vi "DataBase.vi"(7 "udl名称":string="access.udl", 9 "parameters":T1[](array[typedef]), 11 "SQL query":string) -> (1 "recordset data":variant[][](array[variant]))   [LabVIEW 2012]
uses:
  <vilib>/addons/database/Auxilliary.llb/DB Tools Parameter Info.ctl
  <vilib>/addons/database/Auxilliary.llb/DB Tools DataTypes.ctl
  <vilib>/addons/database/Auxilliary.llb/DB Tools Parameter Dir.ctl
  <vilib>/addons/database/Connection.llb/DB Tools Open Connec (Path).vi
  <vilib>/addons/database/Command.llb/Cmd Execute.vi
  <vilib>/addons/database/Recordset.llb/Rec Fetch Recordset Data (CR).vi
  <vilib>/addons/database/Recordset.llb/Rec Destroy - Command.vi
  <vilib>/addons/database/Command.llb/Cmd Delete.vi
  <vilib>/addons/database/NI_Database_API.lvlib
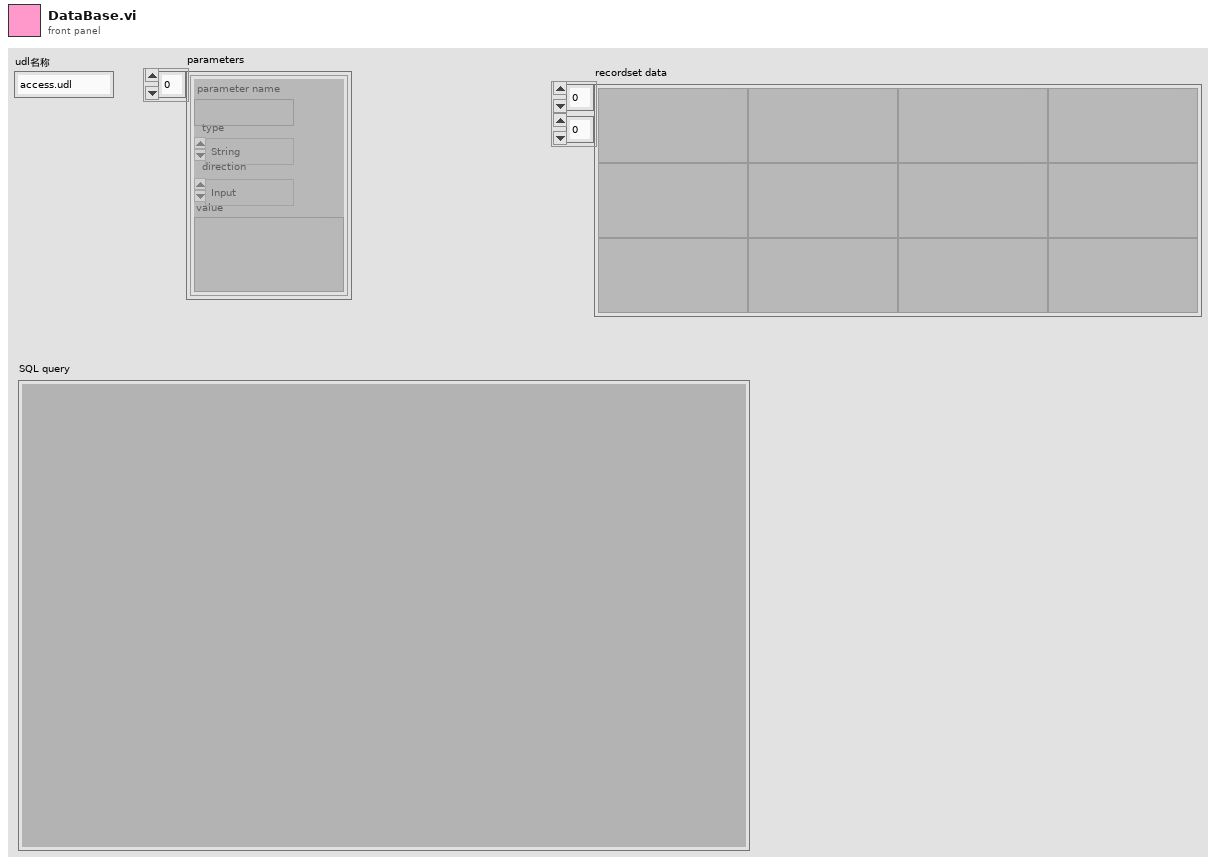
[diagram p1: front panel]
types:
  T1 = typedef "NI_Database_API.lvlib/DB Tools Parameter Info.ctl" = cluster{"parameter name":string, "type":T2, "direction":T3, "value":variant}
  T2 = typedef "NI_Database_API.lvlib/DB Tools DataTypes.ctl" = enum16{"String", "Long (I32)", "Single (SGL)", "Double (DBL)", "Date/Time", "Binary"}
  T3 = typedef "NI_Database_API.lvlib/DB Tools Parameter Dir.ctl" = enum32{"Input", "Output", "Input/Output", "Return Value"}
  T4 = typedef "NI_Database_API.lvlib/Conn ObjectReference.ctl" = refnum<k1>
  T5 = typedef "NI_Database_API.lvlib/Cmd ObjectReference.ctl" = refnum<k1>
  T6 = typedef "NI_Database_API.lvlib/Cmd-Rec Object Reference.ctl" = refnum<k1>
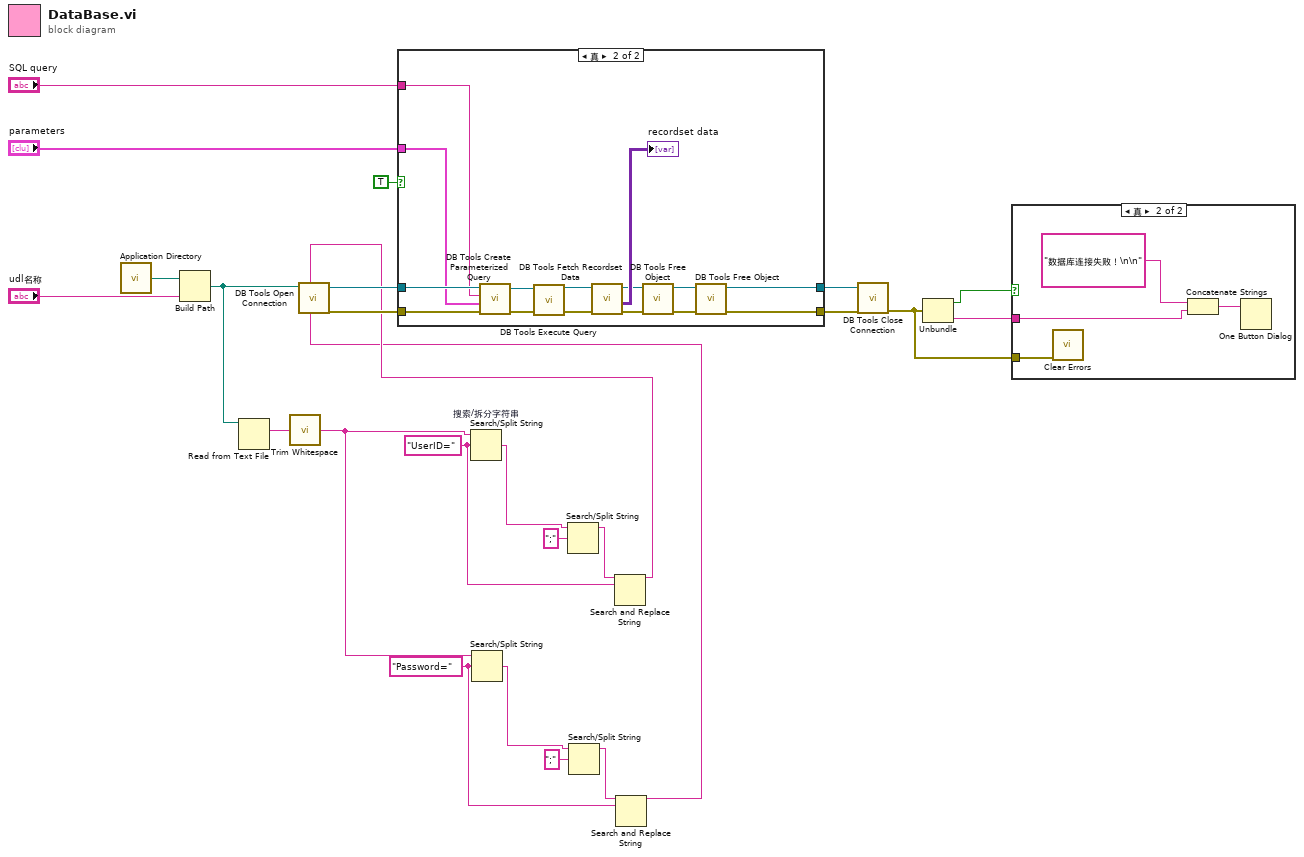
[diagram p0: block diagram]
diagram:
  w10 = "Password=" ("搜索字符串/字符(-)")
  w6 = "UserID=" ("搜索字符串/字符(-)")
  n1 = call <vilib>:"Application Directory.vi"() -> ("Application Directory"=w19:path)
  n2 = Build Path ("创建路径")(base path=w19, name or relative path="udl名称") -> (appended path=w14:path)
  n3 = Read from Text File(file (use dialog)=w14) -> (text=w2:string)  [unwired: 3 in, 3 out]
  n4 = call <vilib>:"Trim Whitespace.vi"("string"=w2) -> ("trimmed string"=w3:string)  [unwired: 1 in]
  n5 = Search/Split String "搜索/拆分字符串"(string=w3, search string/char (-)=w6) -> (match + rest of string=w12:string)  [unwired: 1 in, 2 out]
  n6 = Search/Split String(string=w3, search string/char (-)=w10) -> (match + rest of string=w8:string)  [unwired: 1 in, 2 out]
  n7 = Search/Split String(string=w12, search string/char (-)=";" ("搜索字符串/字符(-)")) -> (substring before match=w11:string)  [unwired: 1 in, 2 out]
  n8 = Search/Split String(string=w8, search string/char (-)=";" ("搜索字符串/字符(-)")) -> (substring before match=w9:string)  [unwired: 1 in, 2 out]
  n9 = Search and Replace String(input string=w11, search string=w6) -> (result string=w5:string)  [unwired: 6 in, 3 out]
  n10 = Search and Replace String(input string=w9, search string=w10) -> (result string=w4:string)  [unwired: 6 in, 3 out]
  n11 = call-poly <vilib>:"DB Tools Open Connection.vi"("password"=w4, "userID"=w5, "connection information"=w14) -> ("error out"=w24:errorcluster, "connection reference"=w25:T4)  [unwired: 5 in]
  n12 = case shown="真" TRUE {
    tunnel: w25 -> [w27 w42]
    tunnel: w24 -> [w26 w41]
    tunnel: "SQL query" -> [_ w40]
    tunnel: [w27 w39] -> w22
    tunnel: [w26 w38] -> w21
    tunnel: "parameters" -> [_ w37]
    frame False {
    }
    frame True {
      n13 = call <vilib>:"DB Tools Create Parameterized Query.vi"("error in (no error)"=w41, "parameters"=w37, "SQL query"=w40, "connection reference"=w42) -> ("error out"=w36:errorcluster, "command reference"=w35:T5)  [unwired: 3 in, 1 out]
      n14 = call-poly <vilib>:"DB Tools Execute Query.vi"("error in (no error)"=w36, "command reference"=w35) -> ("error out"=w28:errorcluster, "command-recordset reference"=w29:T6)  [unwired: 6 in]
      n15 = call-poly <vilib>:"DB Tools Fetch Recordset Data.vi"("error in (no error)"=w28, "command-recordset reference"=w29) -> ("error out"=w31:errorcluster, "recordset data"=→"recordset data":variant[][], "command-recordset reference out"=w30:T6)  [unwired: 3 in]
      n16 = call-poly <vilib>:"DB Tools Free Object.vi"("error in (no error)"=w31, "command-recordset reference"=w30) -> ("error out"=w33:errorcluster, "command reference"=w34:T5)  [unwired: 8 in]
      n17 = call-poly <vilib>:"DB Tools Free Object.vi"("error in (no error)"=w33, "command reference"=w34) -> ("error out"=w38:errorcluster, "connection reference"=w39:T4)  [unwired: 8 in]
    }
  }
  n18 = call <vilib>:"DB Tools Close Connection.vi"("error in (no error)"=w21, "connection reference"=w22) -> ("error out"=w16:errorcluster)  [unwired: 5 in]
  n19 = Unbundle(w16) -> ("status"=w17:bool, "source"=w18:string)  [unwired: 1 out]
  n20 = case shown="真" w17 {
    tunnel: w18 -> [_ w45]
    tunnel: w16 -> [_ w43]
    frame False {
    }
    frame True {
      n21 = call <vilib>:"Clear Errors.vi"("error in (no error)"=w43) -> ()  [unwired: 6 in, 1 out]
      n22 = Concatenate Strings("数据库连接失败！\n\n" ("消息"), w45) -> (w44:string)
      n23 = One Button Dialog(message=w44) -> ()  [unwired: 1 in, 1 out]
    }
  }
